vi "custom_1_stimulus_setup.vi"(1 "input cluster":T1) -> (0 "output cluster":T2)   [LabVIEW 2015]
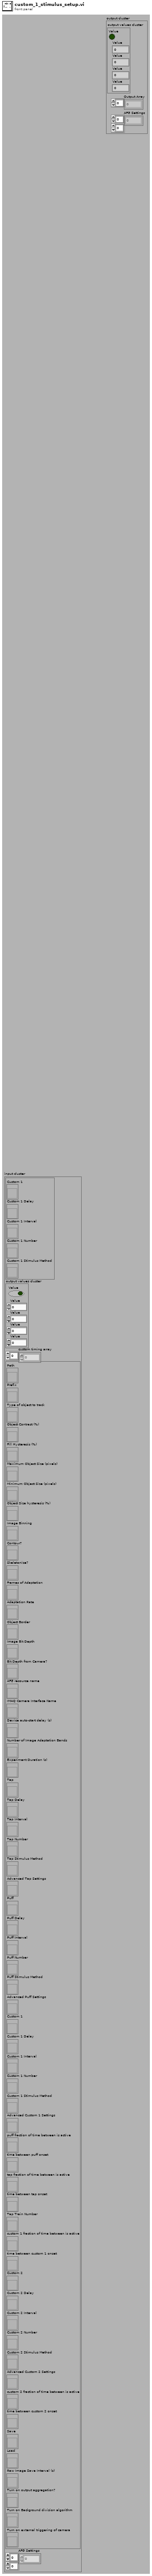
[diagram p1: front panel]
types:
  T1 = cluster{cluster{"Custom 1":refnum<vi>, "Custom 1 Delay":refnum<vi>, "Custom 1 Interval":refnum<vi>, "Custom 1 Number":refnum<vi>, "Custom 1 Stimulus Method":refnum<vi>}, "output values cluster":cluster{"Value":bool, "Value":dbl, "Value":dbl, "Value":dbl, "Value":u16}, "custom timing array":dbl[], cluster{"Path":refnum<vi>, "Prefix":refnum<vi>, "Type of object to track":refnum<vi>, "Object Contrast (%)":refnum<vi>, "Fill Hysteresis (%)":refnum<vi>, "Maximum Object Size (pixels)":refnum<vi>, "Minimum Object Size (pixels)":refnum<vi>, "Object Size hysteresis (%)":refnum<vi>, "Image Binning":refnum<vi>, "Contour?":refnum<vi>, "Skeletonize?":refnum<vi>, "Frames of Adaptation":refnum<vi>, "Adaptation Rate":refnum<vi>, "Object Border":refnum<vi>, "Image Bit Depth":refnum<vi>, "Bit Depth from Camera?":refnum<vi>, "AFG resource name":refnum<vi>, "IMAQ Camera Interface Name":refnum<vi>, "Device auto-start delay (s)":refnum<vi>, "Number of Image Adaptation Bands":refnum<vi>, "Experiment Duration (s)":refnum<vi>, "Tap":refnum<vi>, "Tap Delay":refnum<vi>, "Tap Interval":refnum<vi>, "Tap Number":refnum<vi>, "Tap Stimulus Method":refnum<vi>, "Advanced Tap Settings":refnum<vi>, "Puff":refnum<vi>, "Puff Delay":refnum<vi>, "Puff Interval":refnum<vi>, "Puff Number":refnum<vi>, "Puff Stimulus Method":refnum<vi>, "Advanced Puff Settings":refnum<vi>, "Custom 1":refnum<vi>, "Custom 1 Delay":refnum<vi>, "Custom 1 Interval":refnum<vi>, "Custom 1 Number":refnum<vi>, "Custom 1 Stimulus Method":refnum<vi>, "Advanced Custom 1 Settings":refnum<vi>, "puff fraction of time between is active":refnum<vi>, "time between puff onset":refnum<vi>, "tap fraction of time between is active":refnum<vi>, "time between tap onset":refnum<vi>, "Tap Train Number":refnum<vi>, "custom 1 fraction of time between is active":refnum<vi>, "time between custom 1 onset":refnum<vi>, "Custom 2":refnum<vi>, "Custom 2 Delay":refnum<vi>, "Custom 2 Interval":refnum<vi>, "Custom 2 Number":refnum<vi>, "Custom 2 Stimulus Method":refnum<vi>, "Advanced Custom 2 Settings":refnum<vi>, "custom 2 fraction of time between is active":refnum<vi>, "time between custom 2 onset":refnum<vi>, "Save":refnum<vi>, "Load":refnum<vi>, "Raw Image Save Interval (s)":refnum<vi>, "Turn on output aggregation?":refnum<vi>, "Turn on Background division algorithm":refnum<vi>, "Turn on external triggering of camera":refnum<vi>}, "AFG Settings":dbl[][]}
  T2 = cluster{"output values cluster":cluster{"Value":bool, "Value":dbl, "Value":dbl, "Value":dbl, "Value":u16}, "Output Array":dbl[], "AFG Settings":dbl[][]}
  T3 = cluster{"Custom 1":refnum<vi>, "Custom 1 Delay":refnum<vi>, "Custom 1 Interval":refnum<vi>, "Custom 1 Number":refnum<vi>, "Custom 1 Stimulus Method":refnum<vi>}
  T4 = cluster{"Value":bool, "Value":dbl, "Value":dbl, "Value":dbl, "Value":u16}
  T5 = cluster{"Path":refnum<vi>, "Prefix":refnum<vi>, "Type of object to track":refnum<vi>, "Object Contrast (%)":refnum<vi>, "Fill Hysteresis (%)":refnum<vi>, "Maximum Object Size (pixels)":refnum<vi>, "Minimum Object Size (pixels)":refnum<vi>, "Object Size hysteresis (%)":refnum<vi>, "Image Binning":refnum<vi>, "Contour?":refnum<vi>, "Skeletonize?":refnum<vi>, "Frames of Adaptation":refnum<vi>, "Adaptation Rate":refnum<vi>, "Object Border":refnum<vi>, "Image Bit Depth":refnum<vi>, "Bit Depth from Camera?":refnum<vi>, "AFG resource name":refnum<vi>, "IMAQ Camera Interface Name":refnum<vi>, "Device auto-start delay (s)":refnum<vi>, "Number of Image Adaptation Bands":refnum<vi>, "Experiment Duration (s)":refnum<vi>, "Tap":refnum<vi>, "Tap Delay":refnum<vi>, "Tap Interval":refnum<vi>, "Tap Number":refnum<vi>, "Tap Stimulus Method":refnum<vi>, "Advanced Tap Settings":refnum<vi>, "Puff":refnum<vi>, "Puff Delay":refnum<vi>, "Puff Interval":refnum<vi>, "Puff Number":refnum<vi>, "Puff Stimulus Method":refnum<vi>, "Advanced Puff Settings":refnum<vi>, "Custom 1":refnum<vi>, "Custom 1 Delay":refnum<vi>, "Custom 1 Interval":refnum<vi>, "Custom 1 Number":refnum<vi>, "Custom 1 Stimulus Method":refnum<vi>, "Advanced Custom 1 Settings":refnum<vi>, "puff fraction of time between is active":refnum<vi>, "time between puff onset":refnum<vi>, "tap fraction of time between is active":refnum<vi>, "time between tap onset":refnum<vi>, "Tap Train Number":refnum<vi>, "custom 1 fraction of time between is active":refnum<vi>, "time between custom 1 onset":refnum<vi>, "Custom 2":refnum<vi>, "Custom 2 Delay":refnum<vi>, "Custom 2 Interval":refnum<vi>, "Custom 2 Number":refnum<vi>, "Custom 2 Stimulus Method":refnum<vi>, "Advanced Custom 2 Settings":refnum<vi>, "custom 2 fraction of time between is active":refnum<vi>, "time between custom 2 onset":refnum<vi>, "Save":refnum<vi>, "Load":refnum<vi>, "Raw Image Save Interval (s)":refnum<vi>, "Turn on output aggregation?":refnum<vi>, "Turn on Background division algorithm":refnum<vi>, "Turn on external triggering of camera":refnum<vi>}
  T6 = cluster{"custom 1 fraction of time between is active":refnum<vi>, "time between custom 1 onset":refnum<vi>}
  T7 = cluster{"Custom":refnum<vi>, "Custom Delay":refnum<vi>, "Custom Interval":refnum<vi>, "Custom Number":refnum<vi>, "Custom Stimulus Method":refnum<vi>}
  T8 = cluster{"output values cluster":cluster{"Value":bool, "Value":dbl, "Value":dbl, "Value":dbl, "Value":u16}, "Output Array":dbl[], "Output AFG Settings":dbl[][]}
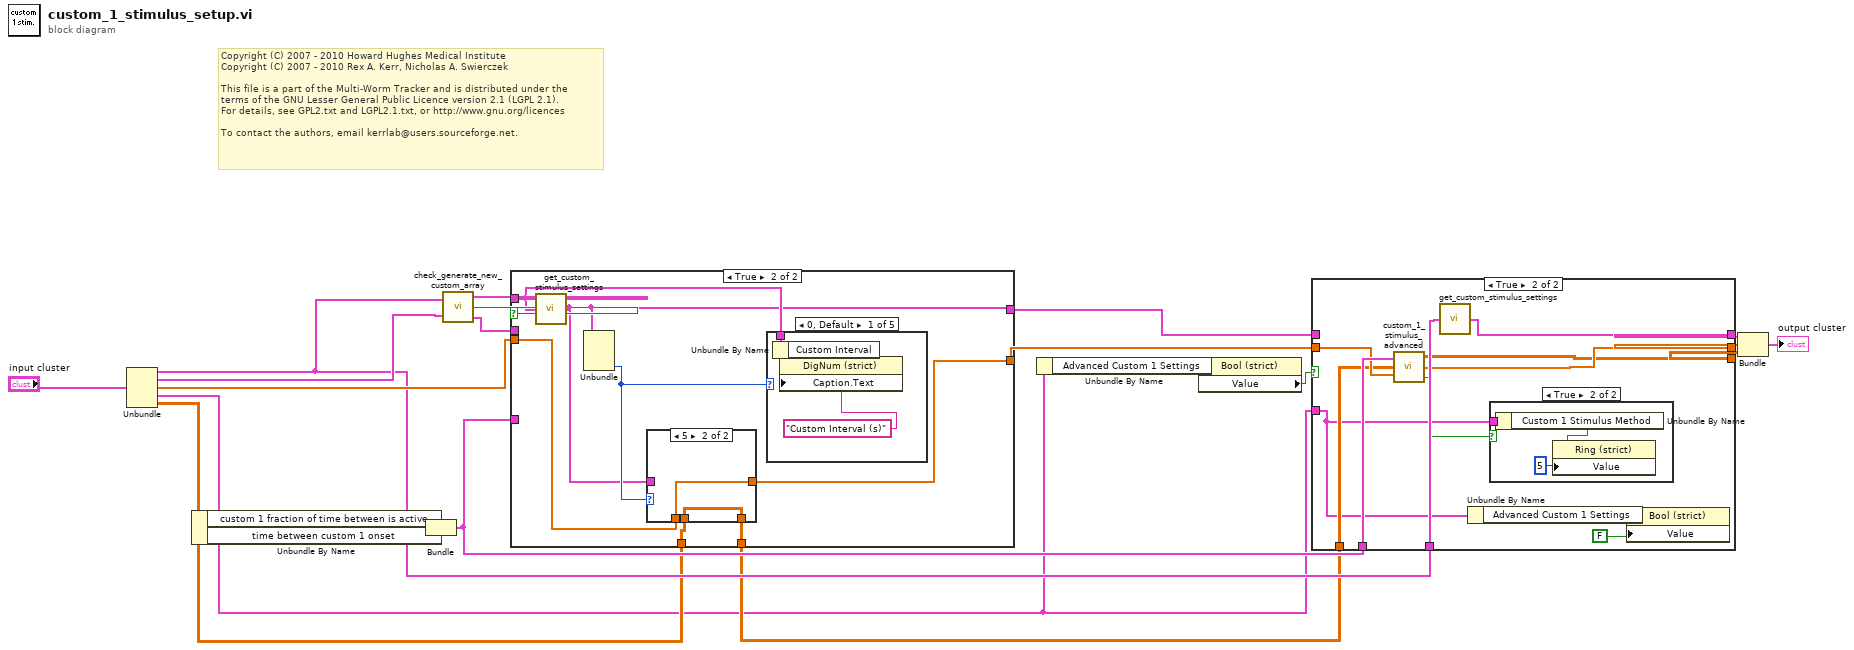
[diagram p0: block diagram]
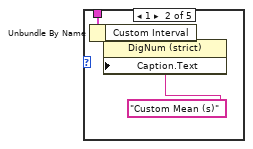
[diagram p5: hidden frame]
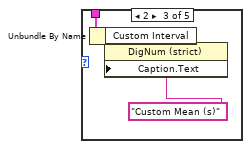
[diagram p6: hidden frame]
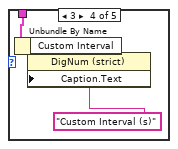
[diagram p7: hidden frame]
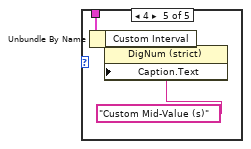
[diagram p8: hidden frame]
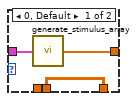
[diagram p9: hidden frame]
diagram:
  # "Copyright (C) 2007 - 2010 Howard Hughes Medical Institute\nCopyright (C) 2007 - 2010 Rex A. Kerr, Nicholas A. Swierczek\n \nThis file is a part of the Multi-Worm Tracker and is distributed under the\nterms of the GNU Lesser General Public Licence version 2.1 (LGPL 2.1).\nFor details, see GPL2.txt and LGPL2.1.txt, or http://www.gnu.org/licences\n \nTo contact the authors, email kerrlab@users.sourceforge.net."
  n1 = Unbundle("input cluster") -> (w8:T3, "output values cluster"=w9:T4, "custom timing array"=w19:dbl[], w3:T5, "AFG Settings"=w7:dbl[][])
  n2 = Unbundle By Name(w3) -> ("custom 1 fraction of time between is active"=w18:refnum<vi>, "time between custom 1 onset"=w17:refnum<vi>)
  n3 = Bundle("custom 1 fraction of time between is active"=w18, "time between custom 1 onset"=w17) -> (w16:T6)  [unwired: 1 in]
  n4 = call "check_generate_new_custom_array.vi"("Cluster"=w8, "output values cluster"=w9) -> ("output cluster"=w12:T7, "Need new custom array?"=w11:bool, "Output values cluster"=w10:T4)
  n5 = case shown="True" w11 {
    tunnel: w12 -> [_ w28]
    tunnel: w10 -> [w24 _]
    tunnel: [w24 w27] -> w20
    tunnel: [w23 w31] -> w21
    tunnel: w19 -> [w23 w30]
    tunnel: w16 -> [_ _]
    tunnel: w7 -> [w22 w26]
    tunnel: [w22 w25] -> w6
    frame False {
    }
    frame True {
      n6 = call "get_custom_stimulus_settings.vi"("input references cluster"=w28) -> ("output values cluster"=w27:T4)
      n7 = Unbundle(w27) -> ("Value"=w29:u16)  [unwired: 4 out]
      n8 = case shown="5" w29 {
        tunnel: [w49 w51] -> w31
        tunnel: w27 -> [w48 _]
        tunnel: w30 -> [_ w51]
        tunnel: w26 -> [w47 w50]
        tunnel: [w47 w50] -> w25
        frame 0, Default {
          n9 = call "generate_stimulus_array.vi"("Values Cluster"=w48) -> ("Array"=w49:dbl[])
        }
        frame 5 {
        }
      }
      n10 = case shown="0, Default" w29 {
        tunnel: w28 -> [w34 w36 w38 w41 w44]
        frame 0, Default {
          n11 = Unbundle By Name(w34) -> ("Custom Interval"=w33:refnum<vi>)
          n12 = property class="DigNum (strict)"(reference=w33, "Caption.Text"="Custom Interval (s)") -> ()  [unwired: 1 in, 2 out]
        }
        frame 1 {
          n13 = Unbundle By Name(w36) -> ("Custom Interval"=w37:refnum<vi>)
          n14 = property class="DigNum (strict)"(reference=w37, "Caption.Text"="Custom Mean (s)") -> ()  [unwired: 1 in, 2 out]
        }
        frame 2 {
          n15 = Unbundle By Name(w38) -> ("Custom Interval"=w40:refnum<vi>)
          n16 = property class="DigNum (strict)"(reference=w40, "Caption.Text"="Custom Mean (s)") -> ()  [unwired: 1 in, 2 out]
        }
        frame 3 {
          n17 = Unbundle By Name(w41) -> ("Custom Interval"=w43:refnum<vi>)
          n18 = property class="DigNum (strict)"(reference=w43, "Caption.Text"="Custom Interval (s)") -> ()  [unwired: 1 in, 2 out]
        }
        frame 4 {
          n19 = Unbundle By Name(w44) -> ("Custom Interval"=w46:refnum<vi>)
          n20 = property class="DigNum (strict)"(reference=w46, "Caption.Text"="Custom Mid-Value (s)") -> ()  [unwired: 1 in, 2 out]
        }
      }
    }
  }
  n21 = Unbundle By Name(w3) -> ("Advanced Custom 1 Settings"=w4:refnum<vi>)
  n22 = property class="Bool (strict)"(reference=w4) -> ("Value"=w2:bool)  [unwired: 1 in, 2 out]
  n23 = case shown="True" w2 {
    tunnel: w21 -> [w54 w61]
    tunnel: [w54 w62] -> w14
    tunnel: w3 -> [_ w56]
    tunnel: w16 -> [_ w63]
    tunnel: w20 -> [w53 _]
    tunnel: [w53 w64] -> w15
    tunnel: w8 -> [_ w65]
    tunnel: w6 -> [w52 w60]
    tunnel: [w52 w59] -> w5
    frame False {
    }
    frame True {
      n24 = call "custom_1_stimulus_advanced.vi"("Input Array"=w61, "Input AFG Settings"=w60, "Cluster"=w63) -> ("x != y?"=w55:bool, "Output Array"=w62:dbl[], "Output AFG Settings"=w59:dbl[][])
      n25 = call "get_custom_stimulus_settings.vi"("input references cluster"=w65) -> ("output values cluster"=w64:T4)
      n26 = Unbundle By Name(w56) -> ("Advanced Custom 1 Settings"=w57:refnum<vi>)
      n27 = case shown="True" w55 {
        tunnel: w56 -> [_ w66]
        frame False {
        }
        frame True {
          n28 = Unbundle By Name(w66) -> ("Custom 1 Stimulus Method"=w67:refnum<vi>)
          n29 = property class="Ring (strict)"(reference=w67, "Value"=u16 5) -> ()  [unwired: 1 in, 2 out]
        }
      }
      n30 = property class="Bool (strict)"(reference=w57, "Value"=FALSE) -> ()  [unwired: 1 in, 2 out]
    }
  }
  n31 = Bundle("output values cluster"=w15, "Output Array"=w14, "Output AFG Settings"=w5) -> (→"output cluster":T8)  [unwired: 1 in]
